vi "PHSensorStart.vi"(0 "Device Info":T1={"Serial Number"=-1, "Channel"=0, "Port"=0}, 1 "Data Interval":i32=-1, 2 "Change Trigger":dbl, 3 "Correction Temperature":dbl=25.0, 11 "error in (no error)":errorcluster, 12 "Connection":u16(ring) items=["No Preference", "Remote", "Local"], 13 "Timeout (mSec)":i32=5000) -> (4 "Phidget ID":u64, 6 "Serial Number Return":i32, 10 "Attached?":bool, 15 "error out":errorcluster)   [LabVIEW 2012, in "Phidget PH Sensor.lvlib"]
doc: "${PHSensor:StartHeader}"
uses:
  <instrlib>/Phidgets/Phidget PH Sensor/Phidget PH Sensor.lvlib
  <instrlib>/Phidgets/Phidget Common/Phidget Common.lvlib
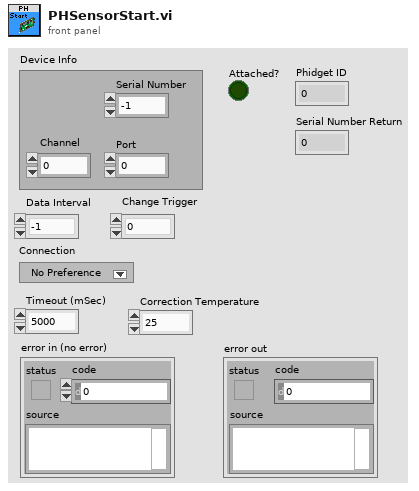
[diagram p1: front panel]
types:
  T1 = cluster{"Serial Number":i32, "Channel":i32, "Port":i32}
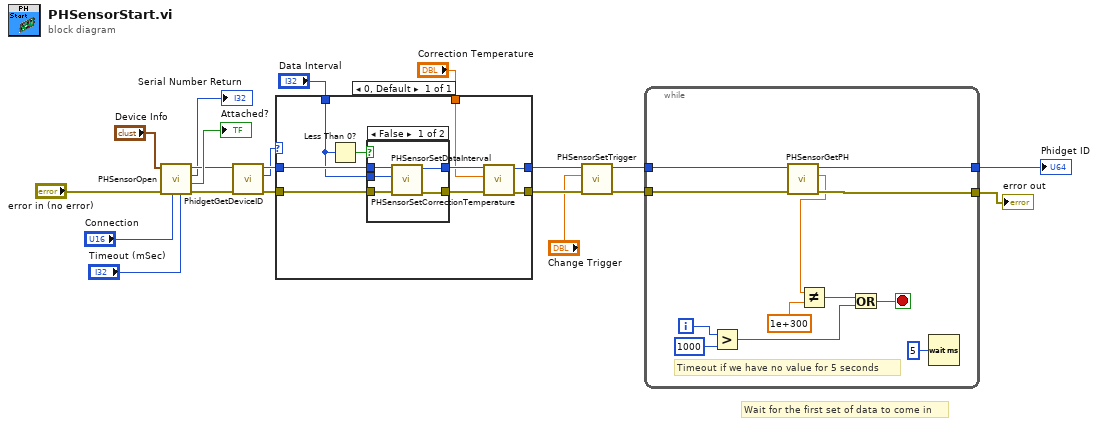
[diagram p0: block diagram]
diagram:
  # "Wait for the first set of data to come in"
  n1 = call <instrlib>:"PHSensorOpen.vi"("Timeout (mSec)"="Timeout (mSec)", "Connection"="Connection", "error in"="error in (no error)", "Device Info"="Device Info") -> ("error out"=w17:errorcluster, "Attached?"=→"Attached?":bool, "Serial Number Return"=→"Serial Number Return":i32, "Phidget ID"=w16:u64)  [unwired: 4 in]
  n2 = call <instrlib>:"PhidgetGetDeviceID.vi"("error in (no error)"=w17, "Device In"=w16) -> ("error out"=w14:errorcluster, "Devie IDs"=w13:u32, "Device Out"=w15:u64)  [unwired: 6 in]
  n3 = case shown="0, Default" w13 {
    tunnel: w14 -> [w28]
    tunnel: [w23] -> w7
    tunnel: w15 -> [w27]
    tunnel: [w22] -> w8
    tunnel: "Data Interval" -> [w26]
    tunnel: "Correction Temperature" -> [w21]
    frame 0, Default {
      n4 = Less Than 0?(x=w26) -> (x < 0?=w29:bool)
      n5 = case shown="False" w29 {
        tunnel: w27 -> [w34 w36]
        tunnel: w28 -> [w32 w35]
        tunnel: [w30 w36] -> w25
        tunnel: [w31 w35] -> w24
        tunnel: w26 -> [w33 _]
        frame False {
          n6 = call <instrlib>:"PHSensorSetDataInterval.vi"("error in (no error)"=w32, "Interval"=w33, "Device In"=w34) -> ("error out"=w31:errorcluster, "Device Out"=w30:u64)  [unwired: 6 in]
        }
        frame True {
        }
      }
      n7 = call <instrlib>:"PHSensorSetCorrectionTemperature.vi"("error in (no error)"=w24, "Temperature"=w21, "Device In"=w25) -> ("error out"=w23:errorcluster, "Device Out"=w22:u64)  [unwired: 6 in]
    }
  }
  n8 = call <instrlib>:"PHSensorSetTrigger.vi"("error in (no error)"=w7, "Trigger"="Change Trigger", "Device In"=w8) -> ("error out"=w9:errorcluster, "Device Out"=w10:u64)  [unwired: 6 in]
  n9 = while {
    tunnel: w10 -> [w46]
    tunnel: w9 -> [w45]
    tunnel: [w43] -> w12
    tunnel: [w44] -> w19
    i -> [w41]
    stop <- w38 stop-if-true
    # "Timeout if we have no value for 5 seconds"
    n10 = Greater?(x=w41, y=1000) -> (0:w39:bool)
    n11 = call <instrlib>:"PHSensorGetPH.vi"("error in (no error)"=w45, "Device In"=w46) -> ("error out"=w44:errorcluster, "pH"=w37:dbl, "Device Out"=w43:u64)  [unwired: 6 in]
    n12 = Not Equal?(x=w37, y=1e+300) -> (x != y?=w40:bool)
    n13 = Or(x=w40, y=w39) -> (x .or. y?=w38:bool)
    n14 = Wait (ms)(milliseconds to wait=u32 5) -> ()  [unwired: 1 out]
  }
  "error out" <- w19
  "Phidget ID" <- w12
